vi "RS-xxx to GPIB ConvBox Factory.vi"(8 "error in (no error)":errorcluster, 10 "settings":T1) -> (0 "error out":errorcluster, 3 "protocol out":refnum<class "Protocol Parent.lvclass">)   [LabVIEW 2018, in "Instrument Addon Scripting API.lvlib"]
doc: "Instantiates a new RS-xxx to GPIB ConvBox Protocol object using the provided RS-xxx to GPIB ConvBox settings."
uses:
  Instrument Addon Scripting API.lvlib
  Addon/Support Libraries/Protocols.lvlibp/RS-xxx to GPIB ConvBox/RS-xxx to GPIB ConvBox Settings.ctl
  Addon/Support Libraries/Protocols.lvlibp/Protocol Parent/Protocol Parent.lvclass
  Addon/Support Libraries/Protocols.lvlibp/RS-xxx to GPIB ConvBox/RS-xxx to GPIB ConvBox.lvclass
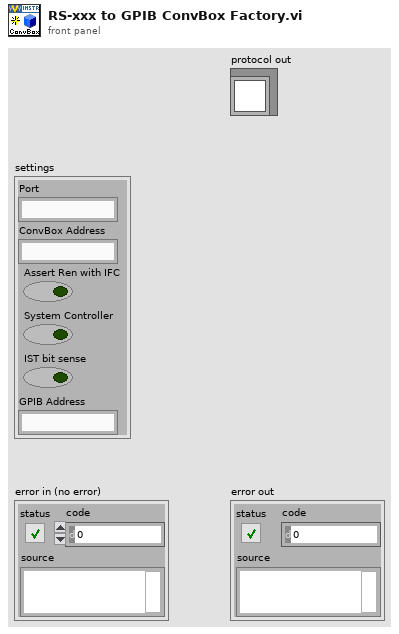
[diagram p1: front panel]
types:
  T1 = typedef "Protocols.lvlibp/RS-xxx to GPIB ConvBox.lvclass/RS-xxx to GPIB ConvBox Settings.ctl" = cluster{"Port":string, "ConvBox Address":string, "Assert Ren with IFC":bool, "System Controller":bool, "IST bit sense":bool, "GPIB Address":string}
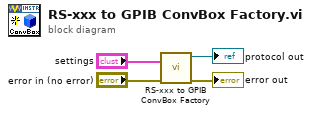
[diagram p0: block diagram]
diagram:
  n1 = call "RS-xxx to GPIB ConvBox Factory.vi"("error in (no error)"="error in (no error)", "RS-xxx to GPIB ConvBox settings"="settings") -> ("error out"=→"error out":errorcluster, "protocol out"=→"protocol out":refnum<class "Protocol Parent.lvclass">)  [unwired: 8 in]
